vi "niRFUtil FWK Object Loader.vi"(8 "error in (no error)":errorcluster, 11 "Option String":string) -> (0 "error out":errorcluster, 3 "Session Out":refnum<class>)   [LabVIEW 2015, in "niRFUtil.lvlib"]
uses:
  niRFUtil.lvlib
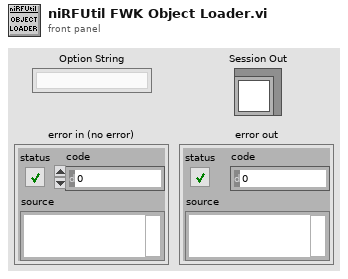
[diagram p1: front panel]
types:
  T1 = typedef "niRFUtil.lvlib/niRFUtil INC FWK Instrument Version Info.ctl" = cluster{"Check Version?":bool, "Instr type":T2, "Major Version":string, "Minor Version":string, "Registry Key":string[], "Product Name":string}
  T2 = typedef "niRFUtil.lvlib/niRFUtil INC FWK Class Types.ctl" = enum16{"RFInstr Agn", "RFSAInstr", "DCPowerInstr"}
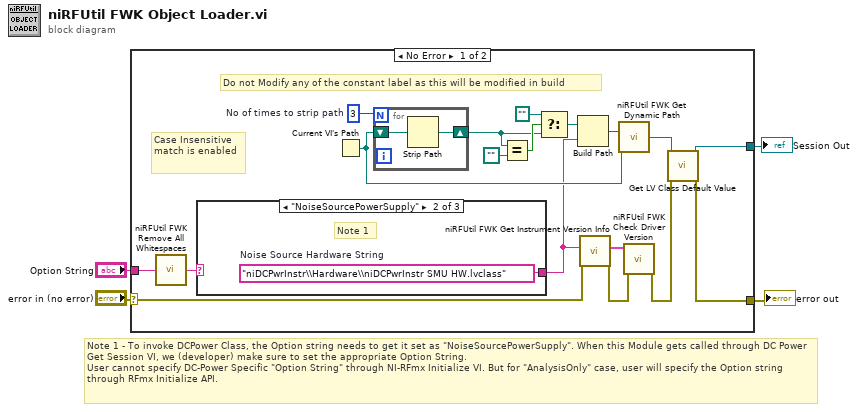
[diagram p0: block diagram]
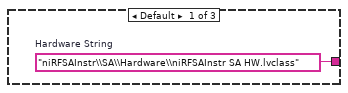
[diagram p2: hidden frame]
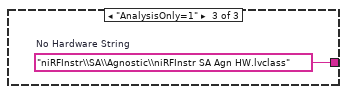
[diagram p3: hidden frame]
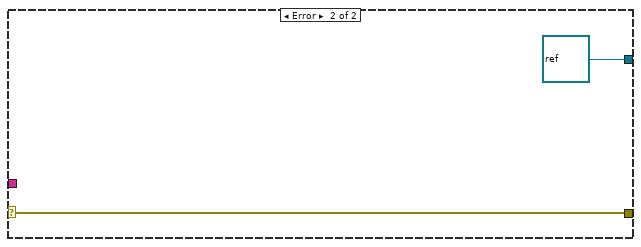
[diagram p4: hidden frame]
diagram:
  # "Note 1 - To invoke DCPower Class, the Option string needs to get it set as \"NoiseSourcePowerSupply\". When this Module gets called through DC Power Get Session VI, we (developer) make sure to set the appropriate Option String. \nUser cannot specify DC-Power Specific \"Option String\" through NI-RFmx Initialize VI. But for \"AnalysisOnly\" case, user will specify the Option string through RFmx Initialize API."
  n1 = case shown="No Error" "error in (no error)" {
    selector: "error in (no error)" -> [w19 w28]
    tunnel: [w22 w28] -> w4
    tunnel: [w21 refnum<class> refnum ("LV Object")] -> w3
    tunnel: "Option String" -> [w20 _]
    frame No Error {
      w18 = 3  # No of times to strip path
      # "Do not Modify any of the constant label as this will be modified in build"
      # "Case Insensitive match is enabled"
      n2 = call "niRFUtil FWK Remove All Whitespaces.vi"("Input String"=w20) -> ("Resultant String"=w9:string)  [unwired: 14 in]
      n3 = case shown="\"NoiseSourcePowerSupply\"" w9 {
        tunnel: [w25 w26 w27] -> w8
        frame Default {
          w25 = "niRFSAInstr\\SA\\Hardware\\niRFSAInstr SA HW.lvclass"  # Hardware String
        }
        frame "NoiseSourcePowerSupply" {
          w26 = "niDCPwrInstr\\Hardware\\niDCPwrInstr SMU HW.lvclass"  # Noise Source Hardware String
          # "Note 1"
        }
        frame "AnalysisOnly=1" {
          w27 = "niRFInstr\\SA\\Agnostic\\niRFInstr SA Agn HW.lvclass"  # No Hardware String
        }
      }
      n4 = Current VI's Path() -> (path=w16:path)
      n5 = for {
        N: w18 -> [_]
        shift-right: [w23] -> w11
        shift-left: w16 -> [w24]
        n6 = Strip Path(path=w24) -> (stripped path=w23:path)  [unwired: 1 out]
      }
      n7 = Equal?(x=w11, y=path "") -> (x = y?=w13:bool)
      n8 = Select(t=path "", s=w13, f=w11) -> (s? t:f=w10:path)
      n9 = Build Path(base path=w10, name or relative path=w8) -> (appended path=w17:path)
      n10 = call "niRFUtil FWK Get Instrument Version Info.vi"("error in (no error)"=w19, "Class Name"=w8) -> ("error out"=w6:errorcluster, "Instr Info"=w7:T1)  [unwired: 8 in]
      n11 = call "niRFUtil FWK Get Dynamic Path.vi"("Virtual Path"=w17, "Current vi Path"=w16) -> ("Actual Path"=w15:path)  [unwired: 13 in]
      n12 = call "niRFUtil FWK Check Driver Version.vi"("error in (no error)"=w6, "Instr Info"=w7) -> ("error out"=w5:errorcluster)  [unwired: 9 in]
      n13 = call <vilib>:"Get LV Class Default Value.vi"("error in (no error)"=w5, "class path"=w15) -> ("error out"=w22:errorcluster, "object"=w21:refnum<class>)  [unwired: 8 in]
    }
    frame Error {
    }
  }
  "error out" <- w4
  "Session Out" <- w3
